vi "ROI group-Generate group number string.vi"(11 "Group number":i32) -> (3 "Group number string":string)   [LabVIEW 2013]
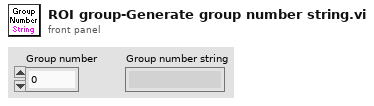
[diagram p1: front panel]
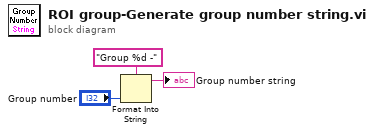
[diagram p0: block diagram]
diagram:
  n1 = Format Into String(format string="Group %d -", "Group number") -> (resulting string=→"Group number string":string)  [unwired: 2 in, 1 out]
